vi "Format Log AI Data.vi"(6 "Sweeping?":bool, 8 "error in (no error)":errorcluster, 10 "waveform":waveform(dbl)[](array[waveform]), 11 "Instrument.Lockin in":refnum<class "Instrument.Lockin.lvclass">) -> (0 "error out":errorcluster, 1 "Log Data":T1[](array[typedef]), 2 "Log Paths":string, 3 "Instrument.Lockin out":refnum<class "Instrument.Lockin.lvclass">, 4 "Times":timestamp[](array[timestamp]))   [LabVIEW 2019, in "Instrument.Lockin.lvlib" / "Instrument.Lockin.lvclass"]
uses:
  Instrument.Lockin.lvclass
  Typedefs/Lockin.LogSweepAOAI--Cluster.ctl
  Instrument.Lockin.lvclass/Instrument.Lockin.ctl
  Generator/Generator.lvclass
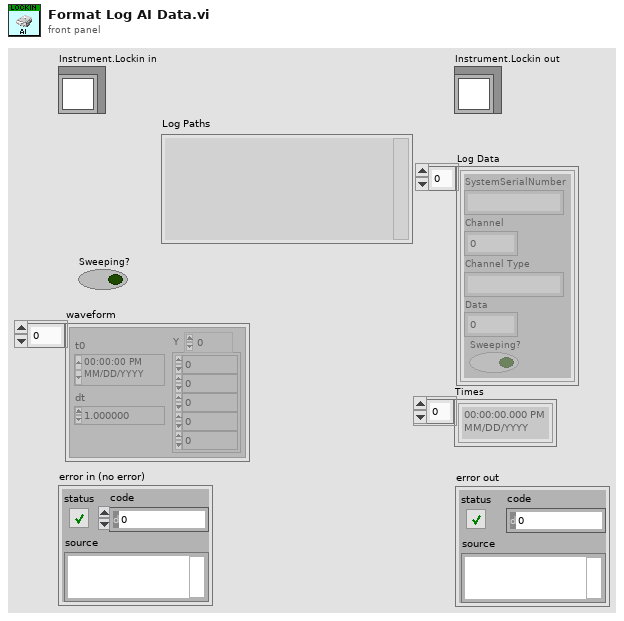
[diagram p1: front panel]
types:
  T1 = typedef "Instrument.Lockin.lvlib/Instrument.Lockin.lvclass/Lockin.LogSweepAOAI--Cluster.ctl" = cluster{"SystemSerialNumber":string, "Channel":i32, "Channel Type":string, "Data":dbl, "Sweeping?":bool}
  T2 = typedef "Instrument.Lockin.lvlib/Instrument.DAQ.lvclass/DeviceInfo--Cluster.ctl" = cluster{"DeviceName":string, "DevIsSimulated":bool, "DeviceSerialNumber":string, "ProductType":string, "ProductCategory":i32, "ProductNumber":u32, "ChassisNumber":u32, "SlotNumber":u32, "ChassisName":string, "ChassisSerialNumber":string, "DevTemp":dbl, "SelfCal.LastDate/Time":string, "SelfCal.LastTemp":dbl, "calibration due?":bool}
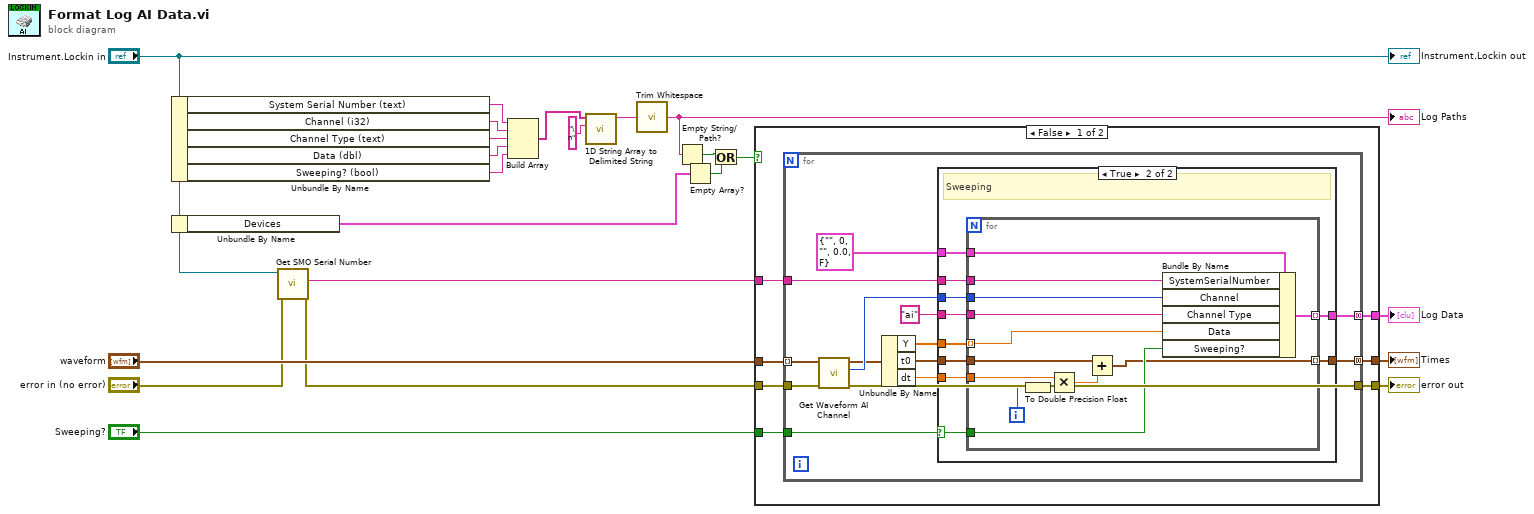
[diagram p0: block diagram]
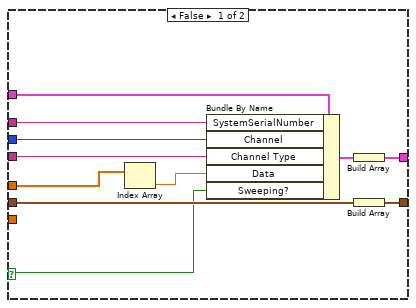
[diagram p2: hidden frame]
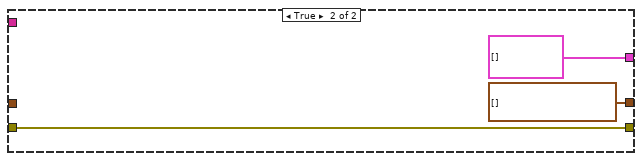
[diagram p3: hidden frame]
diagram:
  n1 = Unbundle By Name("Instrument.Lockin in") -> ("System Serial Number (text)"=w18:string, "Channel (i32)"=w4:string, "Channel Type (text)"=w3:string, "Data (dbl)"=w2:string, "Sweeping? (bool)"=w1:string)
  n2 = Unbundle By Name("Instrument.Lockin in") -> ("Devices"=w6:T2[])
  n3 = call-dynamic "Get SMO Serial Number.vi"("error in (no error)"="error in (no error)", "Instrument.Lockin in"="Instrument.Lockin in") -> ("error out"=w7:errorcluster, "Serial Number"=w9:string)  [unwired: 7 in, 1 out]
  n4 = Build Array(w18, w4, w3, w2, w1) -> (w17:string[])
  n5 = call <vilib>:"1D String Array to Delimited String.vi"("delimiter"="\n", "string array"=w17) -> ("delimited string"=w11:string)  [unwired: 9 in]
  n6 = call <vilib>:"Trim Whitespace.vi"("string"=w11) -> ("trimmed string"=w10:string)  [unwired: 1 in]
  "Log Paths" <- w10
  n7 = Empty String/Path?(string/path=w10) -> (empty?=w13:bool)
  n8 = Empty Array?(array=w6) -> (empty?=w14:bool)
  n9 = Or(x=w13, y=w14) -> (x .or. y?=w12:bool)
  n10 = case shown="False" w12 {
    tunnel: [w29 timestamp[] []] -> w22
    tunnel: [w28 T1[] []] -> w21
    tunnel: "waveform" -> [w27 _]
    tunnel: "Sweeping?" -> [w26 _]
    tunnel: w7 -> [w25 w80]
    tunnel: w9 -> [w24 _]
    tunnel: [w23 w80] -> w15
    frame False {
      n11 = for {
        tunnel: [w43] -> w29 mode=concatenating
        tunnel: [w42] -> w28 mode=concatenating
        tunnel: w24 -> [w41]
        tunnel: w27 -> [w34] mode=indexing
        tunnel: w26 -> [w37]
        tunnel: w25 -> [w35]
        tunnel: [w31] -> w23
        n12 = call "Get Waveform AI Channel.vi"("error in (no error)"=w35, "Reference in"=w34) -> ("error out"=w31:errorcluster, "AI Channel"=w33:i32, "Reference out"=w32:waveform(dbl))  [unwired: 7 in]
        n13 = Unbundle By Name(w32) -> ("Y"=w40:dbl[], "t0"=w38:timestamp, "dt"=w39:dbl)
        n14 = case shown="True" w37 {
          selector: w37 -> [w45 w58]
          tunnel: [w50 w64] -> w43
          tunnel: [w52 w63] -> w42
          tunnel: w41 -> [w51 w62]
          tunnel: w40 -> [w47 w61]
          tunnel: w39 -> [_ w60]
          tunnel: w38 -> [w49 w59]
          tunnel: w33 -> [w48 w57]
          tunnel: T1 {"SystemSerialNumber"="", "Channel"=0, "Channel Type"="", "Data"=0.0, "Sweeping?"=FALSE} ("cluster") -> [w54 w56]
          tunnel: "ai" ("Channel Type") -> [w44 w55]
          frame False {
            n15 = Index Array(array=w47) -> (element=w46:dbl)  [unwired: 1 in]
            n16 = Bundle By Name(cluster=w54, "SystemSerialNumber"=w51, "Channel"=w48, "Channel Type"=w44, "Data"=w46, "Sweeping?"=w45) -> (w53:T1)
            n17 = Build Array(w53) -> (w52:T1[])
            n18 = Build Array(w49) -> (w50:timestamp[])
          }
          frame True {
            # "Sweeping"
            n19 = for {
              tunnel: w59 -> [w73]
              tunnel: w60 -> [w77]
              tunnel: [w65] -> w64 mode=indexing
              tunnel: w61 -> [w72] mode=indexing
              tunnel: w62 -> [w71]
              tunnel: w57 -> [w70]
              tunnel: w58 -> [w69]
              tunnel: [w68] -> w63 mode=indexing
              tunnel: w56 -> [w67]
              tunnel: w55 -> [w66]
              i -> [w76]
              n20 = To Double Precision Float(number=w76) -> (double precision float=w75:dbl)
              n21 = Multiply(x=w77, y=w75) -> (x*y=w74:dbl)
              n22 = Add(x=w73, y=w74) -> (x+y=w65:timestamp)
              n23 = Bundle By Name(cluster=w67, "SystemSerialNumber"=w71, "Channel"=w70, "Channel Type"=w66, "Data"=w72, "Sweeping?"=w69) -> (w68:T1)
            }
          }
        }
      }
    }
    frame True {
    }
  }
  "Times" <- w22
  "Log Data" <- w21
  "error out" <- w15
  "Instrument.Lockin out" <- "Instrument.Lockin in"
